vi "Analog To Digital Conveter.vi"() -> ()   [LabVIEW 2021]
doc: "This VI gives out 1D array of U8 data which contains converted digital data of multiple channels."
uses:
  Controls/Queue Operation.ctl
  Controls/State Cluster.ctl
  Controls/ADC Type.ctl
  Controls/Adc Converter Data.ctl
  Classes/Adc Convertor/Adc Convertor.lvclass
  Controls/Channel Data.ctl
panel:
  out "Error Out":errorcluster
  in  "Error In":errorcluster
  # "Analog To Digital Converter VI"
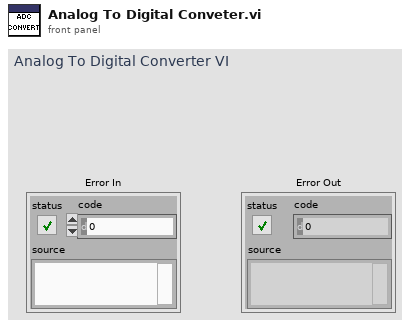
[diagram p1: front panel]
types:
  T1 = typedef "State Cluster.ctl" = cluster{"State":string, "Data":variant}
  T2 = typedef "Queue Operation.ctl" = enum16{"Create", "Enqueue", "Enqueue N", "Enstack", "Dequeue", "Flush", "Release"}
  T3 = typedef "ADC Type.ctl" = cluster{"Channels":string, "Range":dbl, "Resolution":dbl, "Sampling Rate":dbl}
  T4 = typedef "Adc Converter Data.ctl" = cluster{"ADC Type":T3, "Start/Stop":bool, "Start Time":dbl, "U8 Array":u8[], "Sample Rate":dbl, "Channel Number":i32, "Analog Input":dbl, "notifier out":refnum<notifier>, "Adc Convertor Class":refnum<class "Adc Convertor.lvclass">, "Channel Data":T5}
  T5 = typedef "Channel Data.ctl" = cluster{"Channel 1 U8  Array":u8[], "Channel 2 U8  Array ":u8[], "Channel 3 U8  Array":u8[], "Channel 4 U8  Array":u8[]}
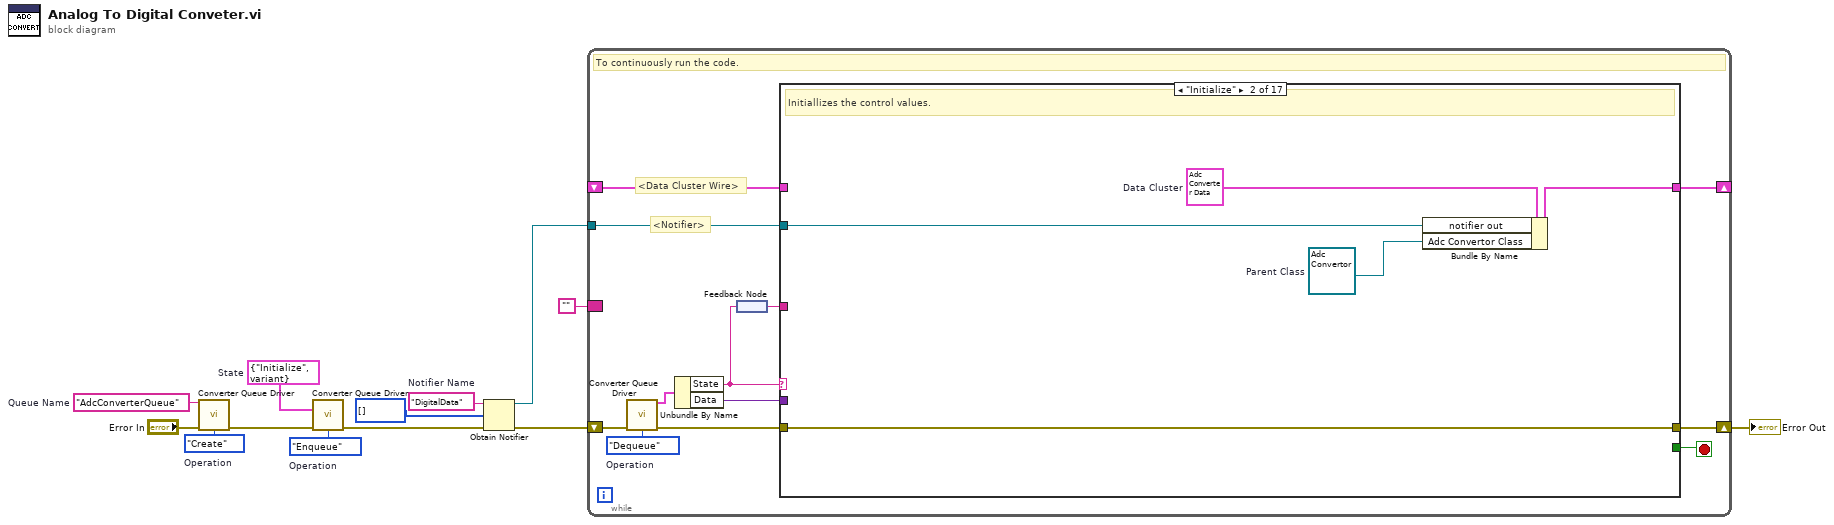
[diagram p0: block diagram]
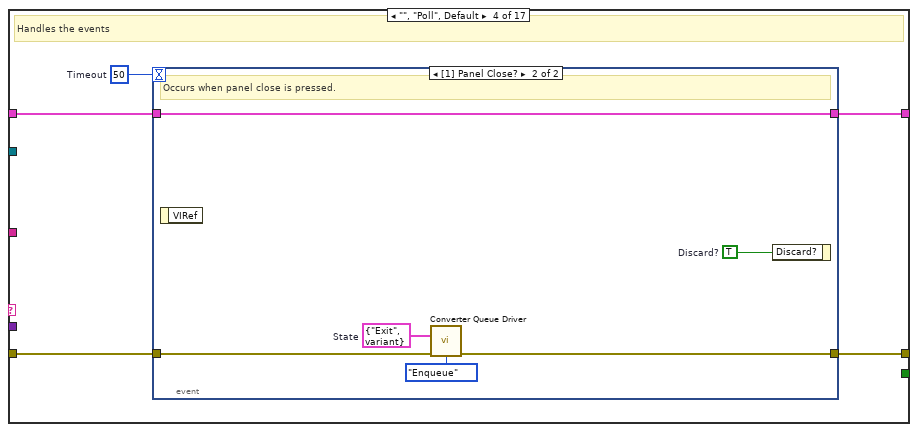
[diagram p4: hidden frame]
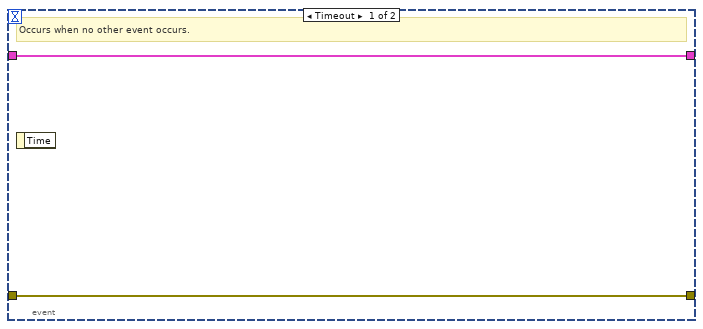
[diagram p5: hidden frame]
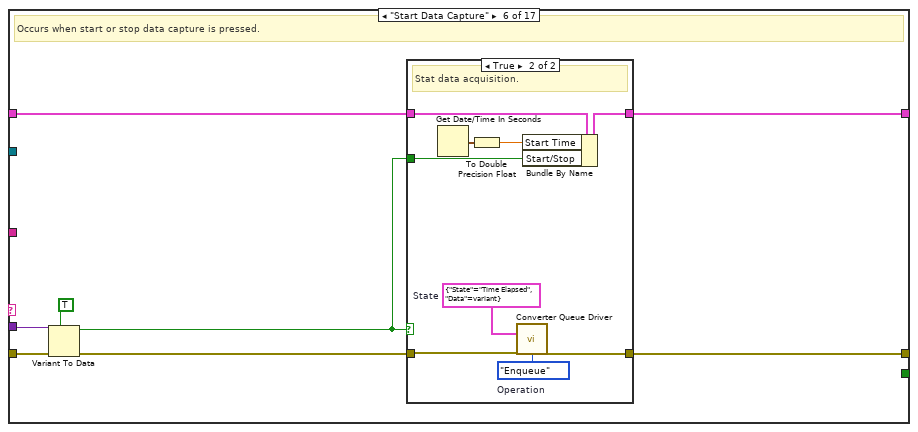
[diagram p7: hidden frame]
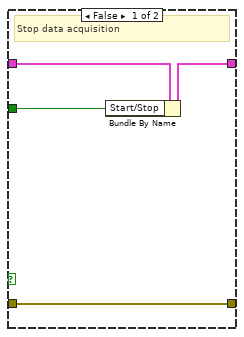
[diagram p8: hidden frame]
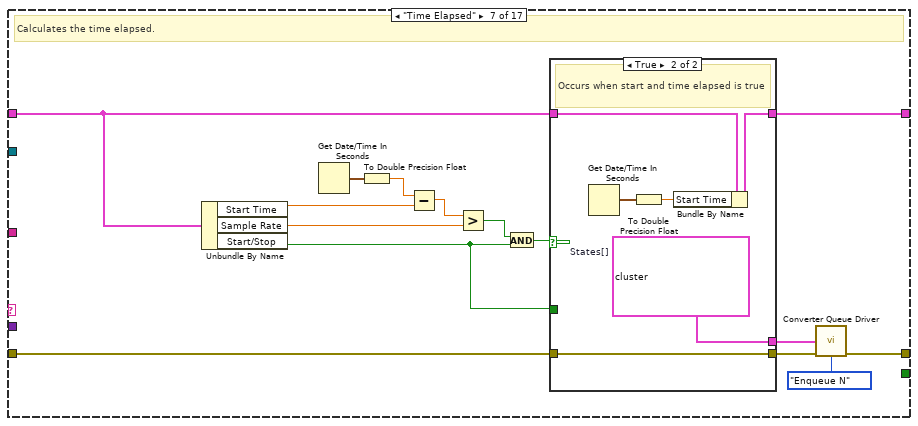
[diagram p9: hidden frame]
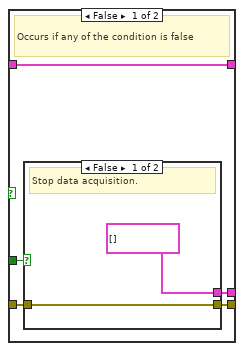
[diagram p10: hidden frame]
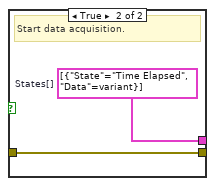
[diagram p11: hidden frame]
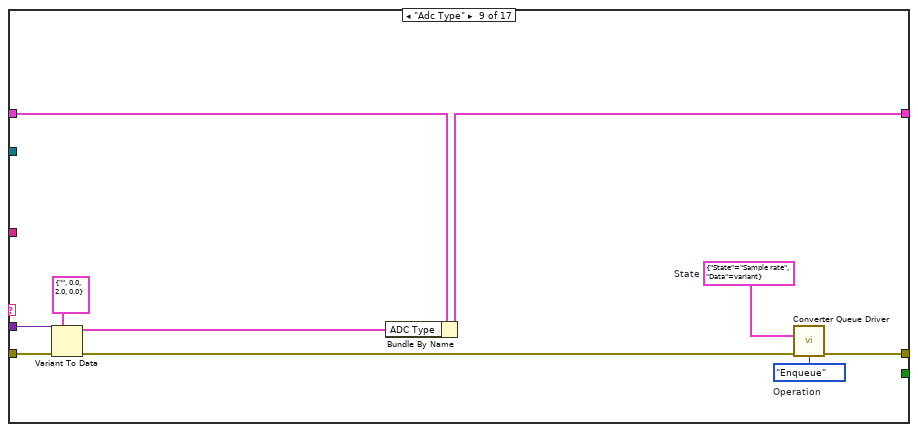
[diagram p13: hidden frame]
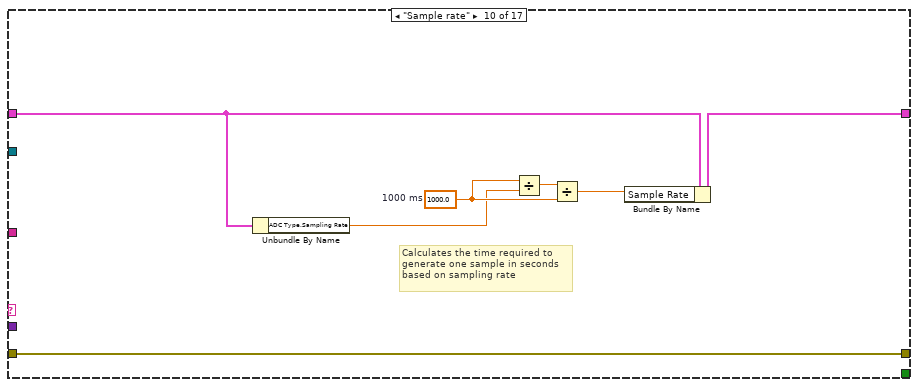
[diagram p14: hidden frame]
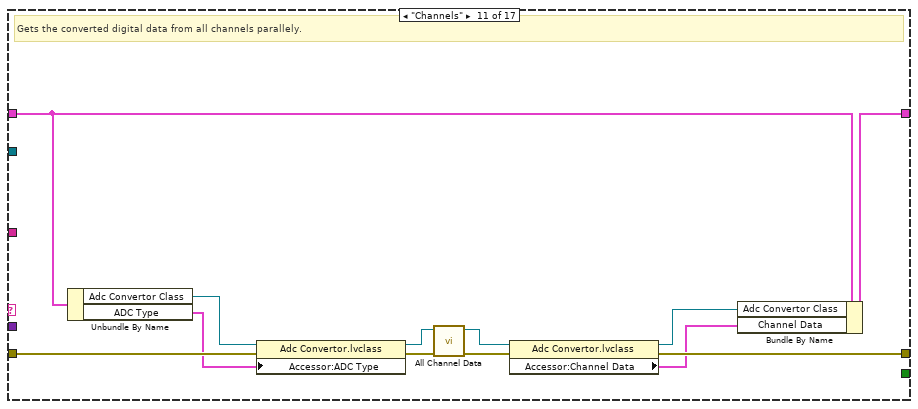
[diagram p15: hidden frame]
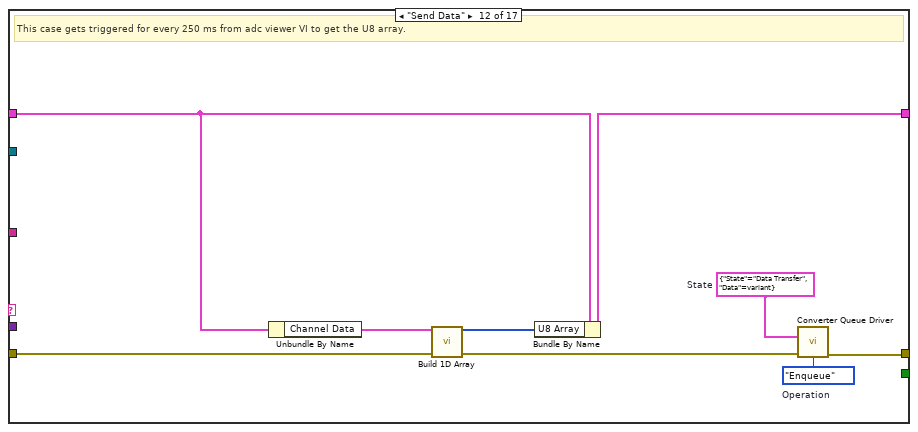
[diagram p16: hidden frame]
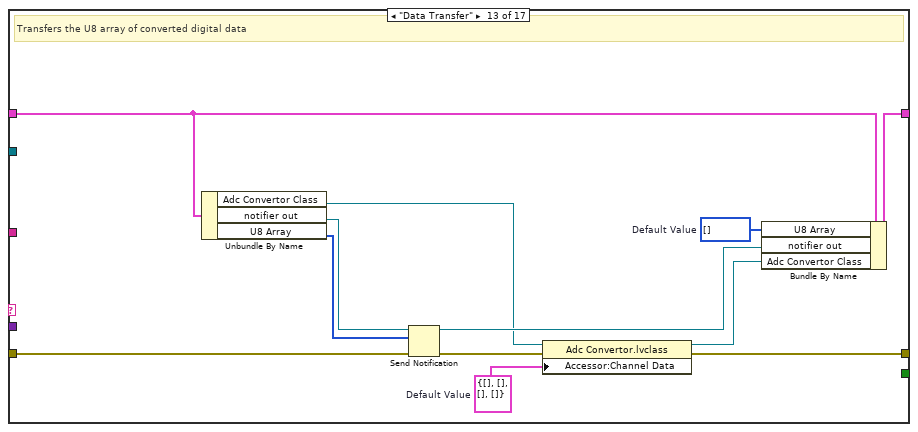
[diagram p17: hidden frame]
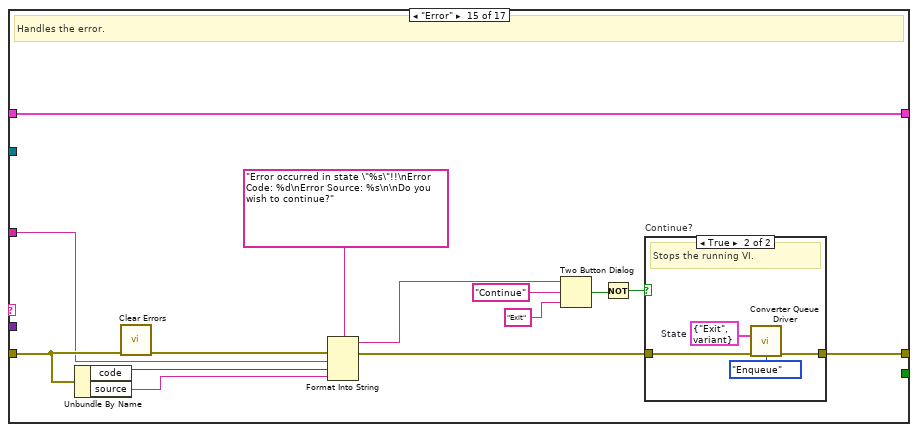
[diagram p19: hidden frame]
diagram:
  w4 = "DigitalData"  # Notifier Name
  w7 = "AdcConverterQueue"  # Queue Name
  w8 = T1 {"State"="Initialize", "Data"=variant}  # State
  w10 = Queue_Operation."Enqueue"  # Operation
  w13 = Queue_Operation."Create"  # Operation
  n1 = call "Converter Queue Driver.vi"("Queue Name"=w7, "error in (no error)"="Error In", "Operation"=w13) -> ("error out"=w11:errorcluster)  [unwired: 11 in, 1 out]
  n2 = call "Converter Queue Driver.vi"("State"=w8, "error in (no error)"=w11, "Operation"=w10) -> ("error out"=w6:errorcluster)  [unwired: 11 in, 1 out]
  n3 = Obtain Notifier(name (unnamed)=w4, notification data type=u8[] [] ("U8 Array"), error in (no error)=w6) -> (notifier out=w2:refnum<notifier>, error out=w5:errorcluster)  [unwired: 1 in, 1 out]
  n4 = while {
    border: "" -> [_]
    shift-right: [w15] -> _
    shift-left: _ -> [w16]
    shift-right: [w18] -> w9
    shift-left: w5 -> [w25]
    tunnel: w2 -> [w14]
    stop <- w17 stop-if-true
    w24 = Queue_Operation."Dequeue"  # Operation
    # "<Notifier>"
    # "<Data Cluster Wire>"
    # "To continuously run the code."
    n5 = call "Converter Queue Driver.vi"("error in (no error)"=w25, "Operation"=w24) -> ("Dequeued Element"=w23:T1, "error out"=w19:errorcluster)  [unwired: 12 in]
    n6 = Unbundle By Name(w23) -> ("State"=w21:string, "Data"=w22:variant)
    n7 = feedback-in #1(w21) -> ()
    n8 = feedback #1() -> (w20:string)
    n9 = case shown="\"Initialize\"" w21 {
      tunnel: w22 -> [_ _ _ _ _ w56 _ _ w111 _ _ _ _ _ _ _ _]
      tunnel: w20 -> [_ _ _ _ _ _ _ _ _ _ _ _ _ _ w158 _ _]
      tunnel: w19 -> [w27 w32 w34 w39 w49 w57 w81 w102 w112 w119 w131 w140 w151 w154 w161 w175 w183]
      tunnel: [w27 w32 w34 w38 w49 w52 w78 w102 w108 w119 w128 w135 w146 w154 w159 w175 w178] -> w18
      tunnel: [_ _ _ _ _ _ _ _ _ _ _ _ _ _ _ _ w180] -> w17
      tunnel: [w26 w31 w33 w36 w48 w51 w79 w101 w104 w117 w130 w138 w147 w153 w155 w174 w177] -> w15
      tunnel: w16 -> [w26 _ w33 w35 w48 w53 w80 w101 w105 w118 w129 w139 w149 w153 w155 w174 w177]
      tunnel: w14 -> [_ w30 _ _ _ _ _ _ _ _ _ _ _ _ _ _ _]
      frame "/****** Initialization *********/" {
        # "Splitter case for initialization."
      }
      frame "Initialize" {
        w28 = T4 {"ADC Type"={"Channels"="", "Range"=0.0, "Resolution"=0.0, "Sampling Rate"=0.0}, "Start/Stop"=FALSE, "Start Time"=0.0, "U8 Array"=[], "Sample Rate"=0.0, "Channel Number"=0, "Analog Input"=0.0, "notifier out"=refnum, "Adc Convertor Class"=refnum, "Channel Data"={"Channel 1 U8  Array"=[], "Channel 2 U8  Array "=[], "Channel 3 U8  Array"=[], "Channel 4 U8  Array"=[]}}  # Data Cluster
        w29 = refnum<class "Adc Convertor.lvclass"> refnum  # Parent Class
        # "Initiallizes the control values."
        n10 = Bundle By Name(cluster=w28, "notifier out"=w30, "Adc Convertor Class"=w29) -> (w31:T4)
      }
      frame "/******** Poll **********/" {
        # "Splitter case for poll."
      }
      frame "", "Poll", Default {
        w37 = 50  # Timeout
        # "Handles the events"
        n11 = event shown="[1] Panel Close?" {
          selector: _ -> [_ _]
          dyn-events: _ -> [_ _]
          timeout: w37 -> [_ _]
          tunnel: w39 -> [w40 w47]
          tunnel: [w40 w46] -> w38
          tunnel: [w41 w42] -> w36
          tunnel: w35 -> [w41 w42]
          event Timeout {
            # "Occurs when no other event occurs."
            n12 = event-data() -> ()  [unwired: 1 in, 1 out]
          }
          event Panel Close? {
            w43 = TRUE  # Discard?
            w44 = T1 {"State"="Exit", "Data"=variant}  # State
            # "Occurs when panel close is pressed."
            n13 = event-data() -> ()  [unwired: 1 in, 1 out]
            n14 = call "Converter Queue Driver.vi"("State"=w44, "error in (no error)"=w47, "Operation"=Queue_Operation."Enqueue") -> ("error out"=w46:errorcluster)  [unwired: 11 in, 1 out]
            n15 = event-data("Discard?"=w43) -> ()  [unwired: 1 in, 1 out]
          }
        }
      }
      frame "/******** Timer Functionalities ********/" {
        # "Splitter case for timer functionalities."
      }
      frame "Start Data Capture" {
        # "Occurs when start or stop data capture is pressed."
        n16 = Variant To Data(error in=w57, type=TRUE, Variant=w56) -> (data=w50:bool, error out=w54:errorcluster)
        n17 = case shown="True" w50 {
          tunnel: w54 -> [w61 w70]
          tunnel: w53 -> [w60 w66]
          tunnel: [w61 w69] -> w52
          tunnel: [w59 w63] -> w51
          tunnel: w50 -> [w58 w62]
          frame False {
            # "Stop data acquisition"
            n18 = Bundle By Name(cluster=w60, "Start/Stop"=w58) -> (w59:T4)
          }
          frame True {
            w67 = T1 {"State"="Time Elapsed", "Data"=variant}  # State
            w68 = Queue_Operation."Enqueue"  # Operation
            # "Stat data acquisition."
            n19 = Get Date/Time In Seconds() -> (seconds since 1Jan1904=w65:timestamp)
            n20 = To Double Precision Float(number=w65) -> (double precision float=w64:dbl)
            n21 = call "Converter Queue Driver.vi"("State"=w67, "error in (no error)"=w70, "Operation"=w68) -> ("error out"=w69:errorcluster)  [unwired: 11 in, 1 out]
            n22 = Bundle By Name(cluster=w66, "Start Time"=w64, "Start/Stop"=w62) -> (w63:T4)
          }
        }
      }
      frame "Time Elapsed" {
        # "Calculates the time elapsed."
        n23 = Unbundle By Name(w80) -> ("Start Time"=w83:dbl, "Sample Rate"=w71:dbl, "Start/Stop"=w72:bool)
        n24 = Get Date/Time In Seconds() -> (seconds since 1Jan1904=w85:timestamp)
        n25 = To Double Precision Float(number=w85) -> (double precision float=w84:dbl)
        n26 = Subtract(x=w84, y=w83) -> (x-y=w82:dbl)
        n27 = Greater?(x=w82, y=w71) -> (0:w73:bool)
        n28 = And(x=w73, y=w72) -> (x .and. y?=w74:bool)
        n29 = case shown="True" w74 {
          tunnel: w81 -> [w88 w100]
          tunnel: [w87 w100] -> w77
          tunnel: w80 -> [w90 w99]
          tunnel: [w90 w98] -> w79
          tunnel: [w89 w95] -> w75
          tunnel: w72 -> [w86 _]
          frame False {
            # "Occurs if any of the condition is false"
            n30 = case shown="False" w86 {
              tunnel: [T1[] [] ("States[]") w94] -> w89
              tunnel: [w92 w93] -> w87
              tunnel: w88 -> [w92 w93]
              frame False {
                # "Stop data acquisition."
              }
              frame True {
                w94 = T1[] [{"State"="Time Elapsed", "Data"=variant}]  # States[]
                # "Start data acquisition."
              }
            }
          }
          frame True {
            w95 = T1[] [{"State"="Channels", "Data"=variant}, {"State"="Time Elapsed", "Data"=variant}]  # States[]
            # "Occurs when start and time elapsed is true"
            n31 = Get Date/Time In Seconds() -> (seconds since 1Jan1904=w96:timestamp)
            n32 = To Double Precision Float(number=w96) -> (double precision float=w97:dbl)
            n33 = Bundle By Name(cluster=w99, "Start Time"=w97) -> (w98:T4)
          }
        }
        n34 = call "Converter Queue Driver.vi"("States[]"=w75, "error in (no error)"=w77, "Operation"=Queue_Operation."Enqueue N") -> ("error out"=w78:errorcluster)  [unwired: 11 in, 1 out]
      }
      frame "/****** Functionalities ********/" {
        # "Splitter case for other functionalities."
      }
      frame "Adc Type" {
        w106 = T1 {"State"="Sample rate", "Data"=variant}  # State
        w107 = Queue_Operation."Enqueue"  # Operation
        n35 = Variant To Data(error in=w112, type=T3 {"Channels"="", "Range"=0.0, "Resolution"=2.0, "Sampling Rate"=0.0} ("ADC Type"), Variant=w111) -> (data=w103:T3, error out=w109:errorcluster)
        n36 = Bundle By Name(cluster=w105, "ADC Type"=w103) -> (w104:T4)
        n37 = call "Converter Queue Driver.vi"("State"=w106, "error in (no error)"=w109, "Operation"=w107) -> ("error out"=w108:errorcluster)  [unwired: 11 in, 1 out]
      }
      frame "Sample rate" {
        w114 = 1000.0  # 1000 ms
        # "Calculates the time required to \ngenerate one sample in seconds\nbased on sampling rate"
        n38 = Unbundle By Name(w118) -> ("ADC Type.Sampling Rate"=w113:dbl)
        n39 = Divide(x=w114, y=w113) -> (x/y=w116:dbl)
        n40 = Divide(x=w116, y=w114) -> (x/y=w115:dbl)
        n41 = Bundle By Name(cluster=w118, "Sample Rate"=w115) -> (w117:T4)
      }
      frame "Channels" {
        # "Gets the converted digital data from all channels parallely."
        n42 = Unbundle By Name(w129) -> ("Adc Convertor Class"=w127:refnum<class "Adc Convertor.lvclass">, "ADC Type"=w120:T3)
        n43 = property class="Adc Convertor.lvclass"(reference=w127, error in=w131, "Accessor:ADC Type"=w120) -> (reference out=w124:refnum<class "Adc Convertor.lvclass">, error out=w126:errorcluster)
        n44 = call "All Channel Data.vi"("Error In"=w126, "Adc Convertor In"=w124) -> ("Error Out"=w125:errorcluster, "Adc Convertor Out"=w123:refnum<class "Adc Convertor.lvclass">)  [unwired: 8 in]
        n45 = property class="Adc Convertor.lvclass"(reference=w123, error in=w125) -> (reference out=w121:refnum<class "Adc Convertor.lvclass">, error out=w128:errorcluster, "Accessor:Channel Data"=w122:T5)
        n46 = Bundle By Name(cluster=w129, "Adc Convertor Class"=w121, "Channel Data"=w122) -> (w130:T4)
      }
      frame "Send Data" {
        w133 = T1 {"State"="Data Transfer", "Data"=variant}  # State
        w134 = Queue_Operation."Enqueue"  # Operation
        # "This case gets triggered for every 250 ms from adc viewer VI to get the U8 array."
        n47 = Unbundle By Name(w139) -> ("Channel Data"=w132:T5)
        n48 = call "Build 1D Array.vi"("Channel Data"=w132, "Error In"=w140) -> ("U8 Array"=w137:u8[], "Error Out"=w136:errorcluster)  [unwired: 12 in]
        n49 = Bundle By Name(cluster=w139, "U8 Array"=w137) -> (w138:T4)
        n50 = call "Converter Queue Driver.vi"("State"=w133, "error in (no error)"=w136, "Operation"=w134) -> ("error out"=w135:errorcluster)  [unwired: 11 in, 1 out]
      }
      frame "Data Transfer" {
        w142 = u8[] []  # Default Value
        w141 = T5 {"Channel 1 U8  Array"=[], "Channel 2 U8  Array "=[], "Channel 3 U8  Array"=[], "Channel 4 U8  Array"=[]}  # Default Value
        # "Transfers the U8 array of converted digital data"
        n51 = Unbundle By Name(w149) -> ("Adc Convertor Class"=w143:refnum<class "Adc Convertor.lvclass">, "notifier out"=w150:refnum<notifier>, "U8 Array"=w144:u8[])
        n52 = Send Notification(notification=w144, notifier=w150, error in (no error)=w151) -> (notifier out=w148:refnum<notifier>, error out=w152:errorcluster)
        n53 = property class="Adc Convertor.lvclass"(reference=w143, error in=w152, "Accessor:Channel Data"=w141) -> (reference out=w145:refnum<class "Adc Convertor.lvclass">, error out=w146:errorcluster)
        n54 = Bundle By Name(cluster=w149, "U8 Array"=w142, "notifier out"=w148, "Adc Convertor Class"=w145) -> (w147:T4)
      }
      frame "/********* Error Handling ********/" {
        # "Splitter case for error handling."
      }
      frame "Error" {
        # "Handles the error."
        n55 = Unbundle By Name(w161) -> ("code"=w157:i32, "source"=w156:string)
        n56 = call <vilib>:"Clear Errors.vi"("error in (no error)"=w161) -> ("error out"=w167:errorcluster)  [unwired: 5 in, 1 out]
        n57 = Format Into String(format string="Error occurred in state \"%s\"!!\nError Code: %d\nError Source: %s\n\nDo you wish to continue?", error in=w167, w158, w157, w156) -> (resulting string=w166:string, error out=w160:errorcluster)  [unwired: 1 in]
        n58 = Two Button Dialog(message=w166, 1:"Exit" ("F button name (\"Cancel\")"), 2:"Continue" ("T button name (\"OK\")")) -> (T button?=w163:bool)
        n59 = Not(x=w163) -> (.not. x?=w162:bool)
        n60 = case "Continue?" shown="True" w162 {
          tunnel: w160 -> [w169 w171]
          tunnel: [w169 w170] -> w159
          frame False {
            # "Continue."
          }
          frame True {
            w172 = T1 {"State"="Exit", "Data"=variant}  # State
            # "Stops the running VI."
            n61 = call "Converter Queue Driver.vi"("State"=w172, "error in (no error)"=w171, "Operation"=Queue_Operation."Enqueue") -> ("error out"=w170:errorcluster)  [unwired: 11 in, 1 out]
          }
        }
      }
      frame "/****** Exit case ********/" {
        # "Splitter case for exiting."
      }
      frame "Exit" {
        w180 = TRUE  # Exit?
        w181 = Queue_Operation."Release"  # Operation
        w182 = Queue_Operation."Flush"  # Operation
        # "Stops the running VI."
        n62 = Unbundle By Name(w177) -> ("notifier out"=w176:refnum<notifier>)
        n63 = call "Converter Queue Driver.vi"("error in (no error)"=w183, "Operation"=w182) -> ("error out"=w184:errorcluster)  [unwired: 12 in, 1 out]
        n64 = call "Converter Queue Driver.vi"("error in (no error)"=w184, "Operation"=w181) -> ("error out"=w179:errorcluster)  [unwired: 12 in, 1 out]
        n65 = Release Notifier(notifier=w176, error in (no error)=w179) -> (error out=w178:errorcluster)  [unwired: 1 in, 2 out]
      }
    }
  }
  "Error Out" <- w9
